vi "Load DAQmx Insruments.vi"() -> (3 "Instruments":refnum<class "Dynamic Instrument.lvclass">[](array[class]))   [LabVIEW 2016]
uses:
  Dynamic Instrument/Dynamic Instrument/Dynamic Instrument.lvclass
  DAQmx Digitizer/DAQmx Digitizer.lvclass
  C:/github/NHMFL_Core/Libraries/NI-DAQ/Dynamic Load/Dynamic Instrument/Dynamic Instrument/Dynamic Instrument.lvclass
  Dynamic Instrument/Dynamic Instrument/Dynamic Instrument.lvclass/Dynamic Instrument.ctl
  Dynamic Instrument/Dynamic Instrument/Write Instrument Name.vi
  <resource>/objmgr/daqmx.rc
panel:
  out "path":path
  out "Device names":tag[](array[tag])
  out "Error Out":errorcluster
  in  "Error In":errorcluster
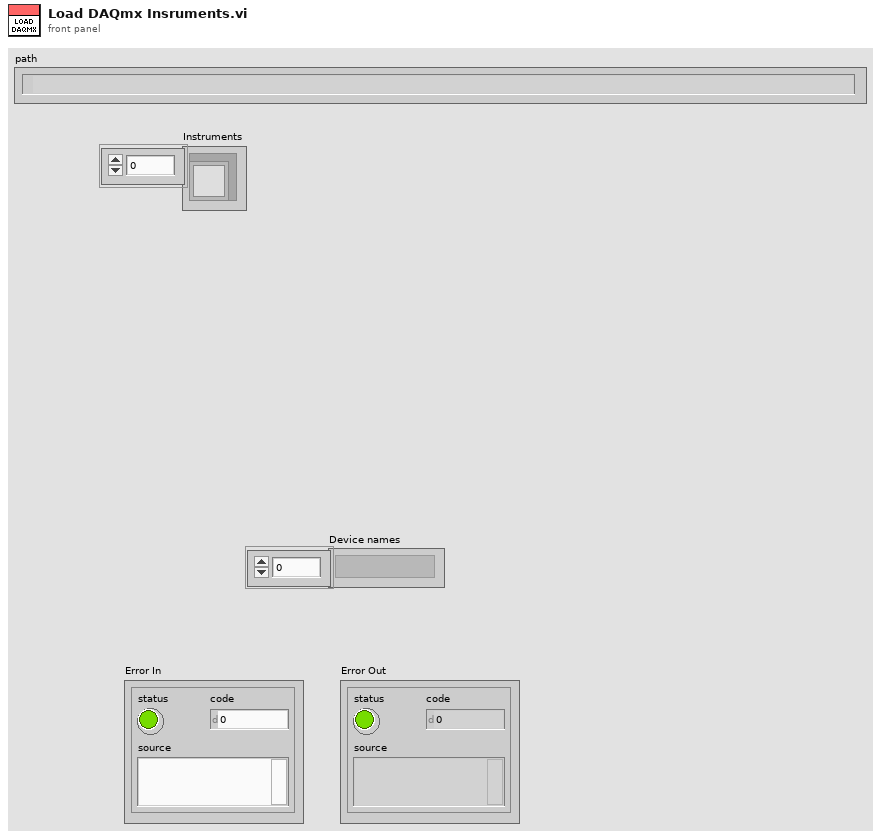
[diagram p1: front panel]
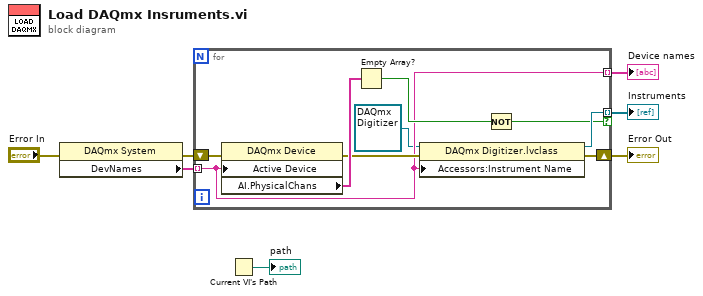
[diagram p0: block diagram]
diagram:
  n1 = property class="DAQmx System"(error in="Error In") -> (error out=w6:errorcluster, "DevNames"=w7:tag[])  [unwired: 1 in, 1 out]
  n2 = for {
    tunnel: w7 -> [w9] mode=indexing
    shift-right: [w13] -> w4
    shift-left: w6 -> [w16]
    tunnel: [w12] -> w2 mode=indexing if=w10
    tunnel: [w9] -> w3 mode=indexing
    n3 = property class="DAQmx Device"(error in=w16, "Active Device"=w9) -> (error out=w14:errorcluster, "AI.PhysicalChans"=w15:tag[])  [unwired: 1 in, 1 out]
    n4 = Empty Array?(array=w15) -> (empty?=w11:bool)
    n5 = property class="DAQmx Digitizer.lvclass"(reference=refnum<class "DAQmx Digitizer.lvclass"> refnum ("DAQmx Digitizer.lvlib:DAQmx Digitizer.lvclass"), error in=w14, "Accessors:Instrument Name"=w9) -> (reference out=w12:refnum<class "DAQmx Digitizer.lvclass">, error out=w13:errorcluster)
    n6 = Not(x=w11) -> (.not. x?=w10:bool)
  }
  "Instruments" <- w2
  "Error Out" <- w4
  "Device names" <- w3
  n7 = Current VI's Path() -> (path=→"path":path)
